vi "Post Media Tweet - From LabVIEW Picture Type.vi"(8 "error in":errorcluster, 9 "LabVIEW Picture Type":picture, 10 "Tweet":string, 11 "Twitter Handle In":T1={"OAuth Credentials"={"Signature Method"=enum."HMAC-SHA1", "Version"="1.0", "Client"={"Token"="", "Secret"=""}, "Access"={"Token"="", "Secret"=""}}, "since ID"="", "max ID"="", "Screen Name"=""}) -> (0 "error out":errorcluster, 3 "Twitter Handle Out":T1={"OAuth Credentials"={"Signature Method"=enum."HMAC-SHA1", "Version"="1.0", "Client"={"Token"="", "Secret"=""}, "Access"={"Token"="", "Secret"=""}}, "since ID"="", "max ID"="", "Screen Name"=""})   [LabVIEW 2011, in "i3-twitter.lvlib"]
doc: "Posts a status update as a Tweet for the authenticated user that includes a picture file in the LabVIEW Picture Type format. Duplicate posts will result in an error message from Twitter."
uses:
  i3-twitter.lvlib
  Controls/Twitter Handle.ctl
  i3-oauth/Controls/OAuth Handle.ctl
  i3-oauth/Controls/Signature Method.ctl
  i3-oauth/Controls/Credentials.ctl
  <vilib>/httpClient/MultipartData.ctl
  i3-oauth/Controls/HTTP Method.ctl
  i3-oauth/i3-oauth.lvlib
  <vilib>/httpClient/LabVIEWHTTPClient.lvlib
  Libs/i3-twitter-lvpng.llb/i3-twitter-lvpng.lvlib
panel:
  out "headers (response)":string
  out "body (response)":string
  out "Header Value":string
  out "Full URL":string
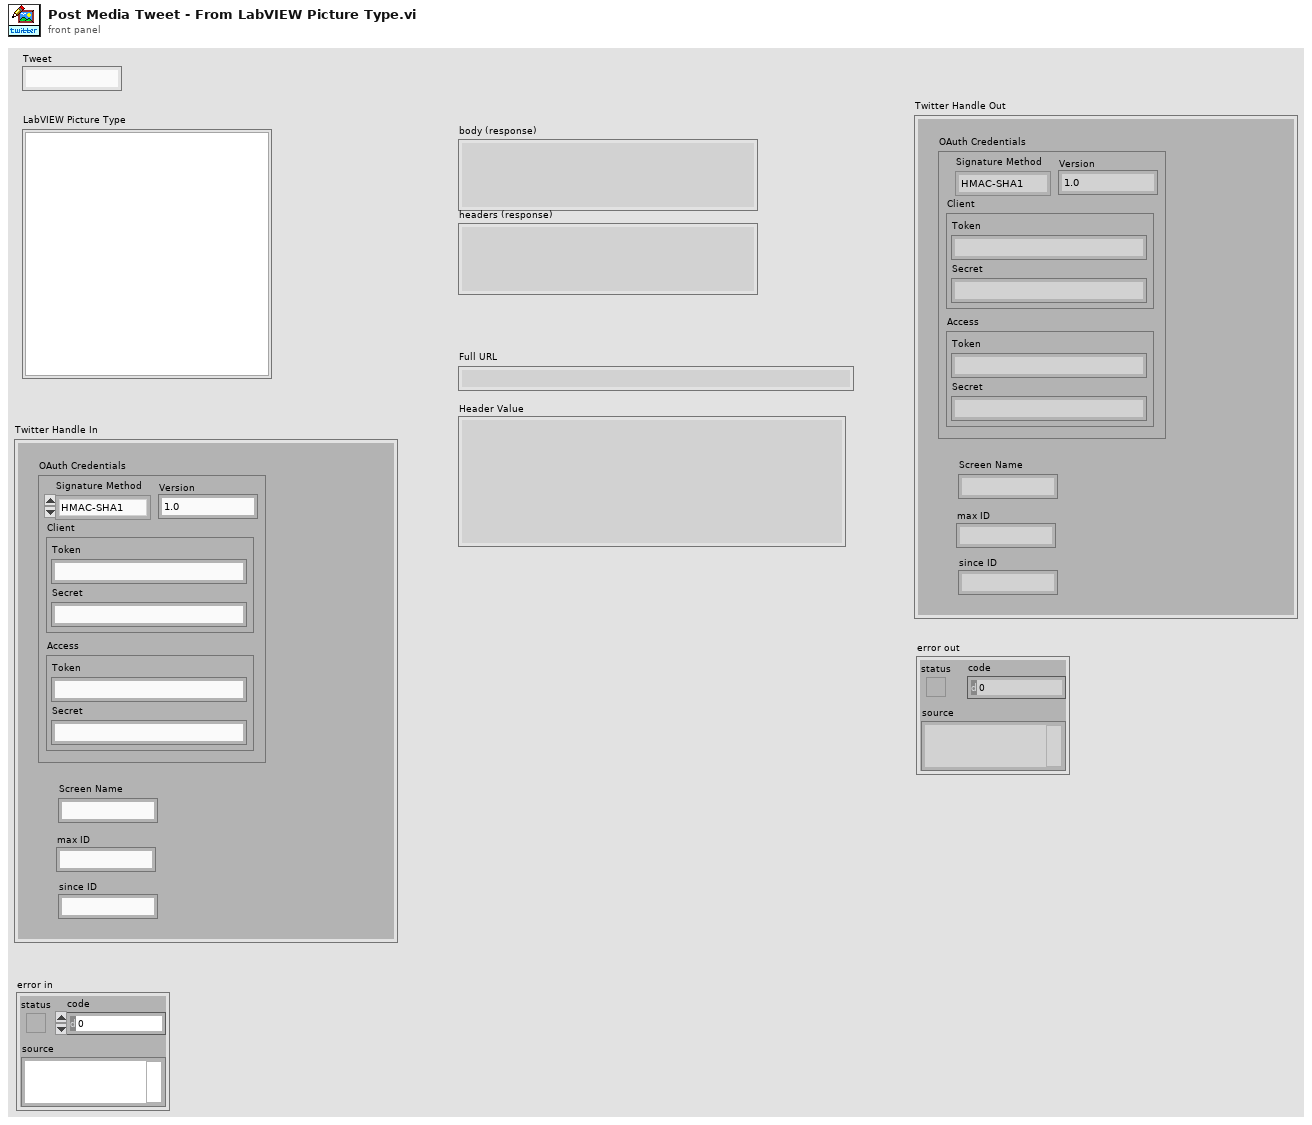
[diagram p1: front panel]
types:
  T1 = typedef "i3-twitter.lvlib/Twitter Handle.ctl" = cluster{"OAuth Credentials":T2, "since ID":string, "max ID":string, "Screen Name":string}
  T2 = typedef "i3-oauth.lvlib/OAuth Handle.ctl" = cluster{"Signature Method":T3, "Version":string, "Client":T4, "Access":T4}
  T3 = typedef "i3-oauth.lvlib/Signature Method.ctl" = enum16{"HMAC-MD5", "HMAC-SHA1", "HMAC-SHA224", "HMAC-SHA256", "HMAC-SHA384", "HMAC-SHA512"}
  T4 = typedef "i3-oauth.lvlib/Credentials.ctl" = cluster{"Token":string, "Secret":string}
  T5 = typedef "LabVIEWHTTPClient.lvlib/MultipartData.ctl" = cluster{"Name":string, "Value":string, "File":path, "Filename":string, "MIME type":string}
  T6 = typedef "i3-oauth.lvlib/HTTP Method.ctl" = enum16{"GET", "POST", "PUT", "DELETE"}
  T7 = typedef "imagedata.ctl" = cluster{"image type":i32, "image depth":i32, "image":u8[], "mask":u8[], "colors":u32[], "Rectangle":cluster{"left":i16, "top":i16, "right":i16, "bottom":i16}}
  T8 = cluster{"left":i16, "top":i16, "right":i16, "bottom":i16}
  T9 = typedef "LabVIEWHTTPClient.lvlib/ClientHandle.ctl" = refnum<k1>
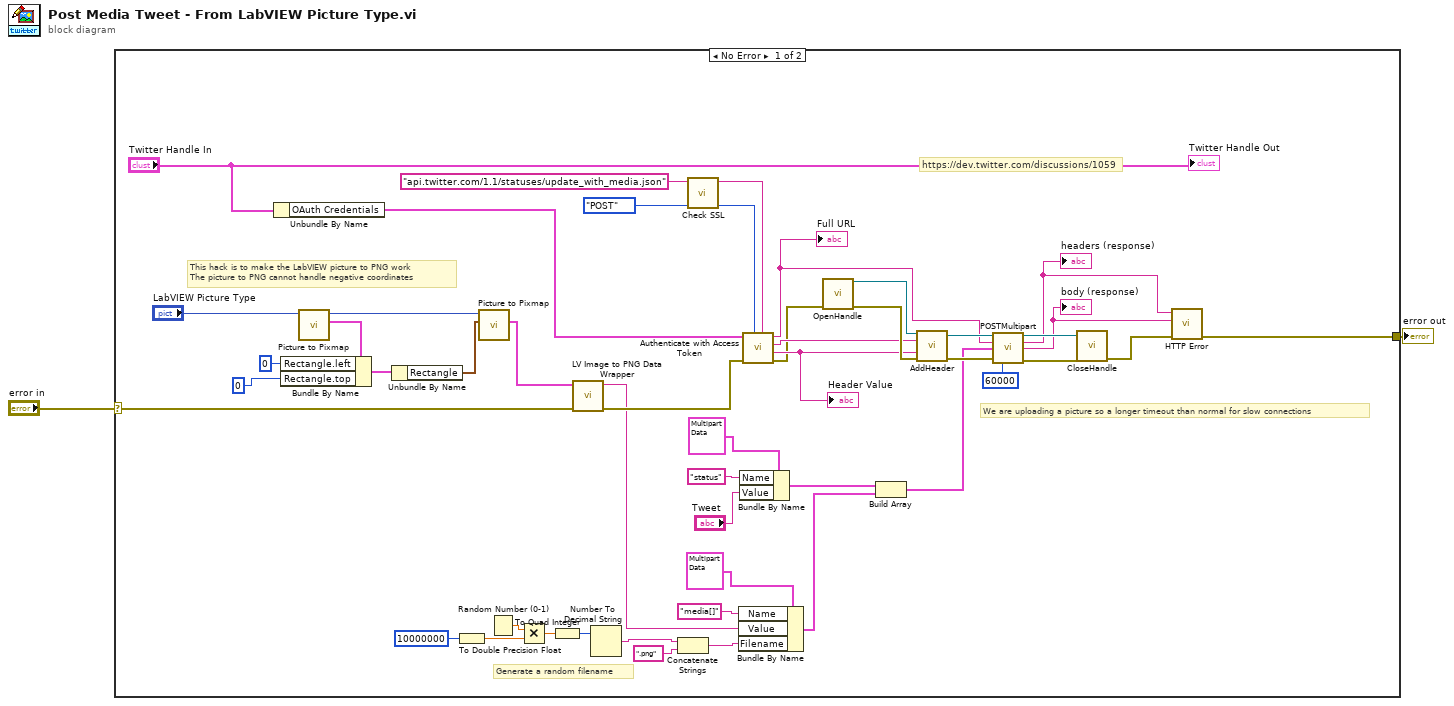
[diagram p0: block diagram]
diagram:
  n1 = case shown="No Error" "error in" {
    selector: "error in" -> [w10 w50]
    tunnel: [w12 w50] -> w2
    frame No Error {
      # "We are uploading a picture so a longer timeout than normal for slow connections"
      # "Generate a random filename"
      # "This hack is to make the LabVIEW picture to PNG work\nThe picture to PNG cannot handle negative coordinates"
      # "https://dev.twitter.com/discussions/1059"
      n2 = Unbundle By Name("Twitter Handle In") -> ("OAuth Credentials"=w6:T2)
      n3 = call <vilib>:"Picture to Pixmap.vi"("picture"="LabVIEW Picture Type") -> ("image data"=w27:T7, "new picture"=w31:picture)  [unwired: 9 in]
      n4 = Bundle By Name(cluster=w27, "Rectangle.left"=i16 0, "Rectangle.top"=i16 0) -> (w30:T7)
      n5 = Unbundle By Name(w30) -> ("Rectangle"=w32:T8)
      n6 = To Double Precision Float(number=10000000) -> (double precision float=w24:dbl)
      n7 = call <vilib>:"Picture to Pixmap.vi"("rect"=w32, "picture"=w31) -> ("image data"=w7:T7)  [unwired: 8 in, 1 out]
      n8 = Random Number (0-1)() -> (number: 0 to 1=w26:dbl)
      n9 = Multiply(x=w26, y=w24) -> (x*y=w15:dbl)
      n10 = To Quad Integer(1:w15) -> (0:w14:i64)
      n11 = call "LV Image to PNG Data Wrapper.vi"("error in (no error)"=w10, "image data"=w7) -> ("error out"=w9:errorcluster, "png data"=w8:string)  [unwired: 8 in]
      n12 = Number To Decimal String(number=w14) -> (decimal integer string=w18:string)  [unwired: 1 in]
      n13 = Concatenate Strings(w18, ".png" ("string")) -> (w16:string)
      n14 = call "Check SSL.vi"("Input URL"="api.twitter.com/1.1/statuses/update_with_media.json" ("Base URL")) -> ("Output URL"=w4:string)  [unwired: 8 in]
      n15 = Bundle By Name(cluster=T5 {"Name"="", "Value"="", "File"=path "", "Filename"="", "MIME type"="application/octet-stream"} ("Element"), "Name"="media[]", "Value"=w8, "Filename"=w16) -> (w35:T5)
      n16 = Bundle By Name(cluster=T5 {"Name"="", "Value"="", "File"=path "", "Filename"="", "MIME type"="application/octet-stream"} ("Element"), "Name"="status", "Value"="Tweet") -> (w39:T5)
      n17 = call "Authenticate with Access Token.vi"("Base URL"=w4, "HTTP Method"=HTTP_Method."POST", "error in (no error)"=w9, "OAuth Handle"=w6) -> ("error out"=w13:errorcluster, "Header Value"=w46:string, "Header Parameter"=w47:string, "Full URL"=w41:string)  [unwired: 3 in, 1 out]
      "Full URL" <- w41
      "Header Value" <- w46
      n18 = call <vilib>:"OpenHandle.vi"("error in (no error)"=w13) -> ("client handle out"=w49:T9, "error out"=w48:errorcluster)  [unwired: 13 in]
      n19 = Build Array(w39, w35) -> (w38:T5[])
      n20 = call <vilib>:"AddHeader.vi"("client handle"=w49, "header"=w47, "value"=w46, "error in (no error)"=w48) -> ("client handle out"=w45:T9, "error out"=w44:errorcluster)  [unwired: 10 in]
      n21 = call <vilib>:"POSTMultipart.vi"("client handle"=w45, "url"=w41, "data"=w38, "error in (no error)"=w44, "timeout (10000)"=60000) -> ("client handle out"=w42:T9, "headers"=w19:string, "body"=w20:string, "error out"=w43:errorcluster)  [unwired: 7 in]
      "body (response)" <- w20
      "headers (response)" <- w19
      n22 = call <vilib>:"CloseHandle.vi"("client handle"=w42, "error in (no error)"=w43) -> ("error out"=w21:errorcluster)  [unwired: 13 in]
      n23 = call "HTTP Error.vi"("error in (no error)"=w21, "Body"=w20, "Header"=w19) -> ("error out"=w12:errorcluster)  [unwired: 6 in, 2 out]
      "Twitter Handle Out" <- "Twitter Handle In"
    }
    frame Error {
    }
  }
  "error out" <- w2
